vi "CatchSteer.vi"(6 "isOmni":bool, 8 "DefY":dbl, 9 "DefX":dbl, 10 "ReInit":bool) -> (0 "Translation X":dbl, 1 "Translation Y":dbl)   [LabVIEW 2013]
uses:
  Common Code/Change Detect Boolean.vi
  Robot Global Data.vi
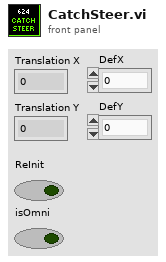
[diagram p1: front panel]
types:
  T1 = typedef "Vision Packet.ctl" = cluster{"Ball Found?":bool, "Ball X":dbl, "Ball Y":dbl, "Ball Diameter":dbl, "Gyro":dbl, "Vision Target":T2, "Timestamp":u32, "Camera":i16}
  T2 = typedef "Goal Info.ctl" = cluster{"Found?":bool, "Target Center":cluster{"X":dbl, "Y":dbl}, "Distance (ft)":dbl, "Hot?":bool, "Width":dbl, "Left?":bool}
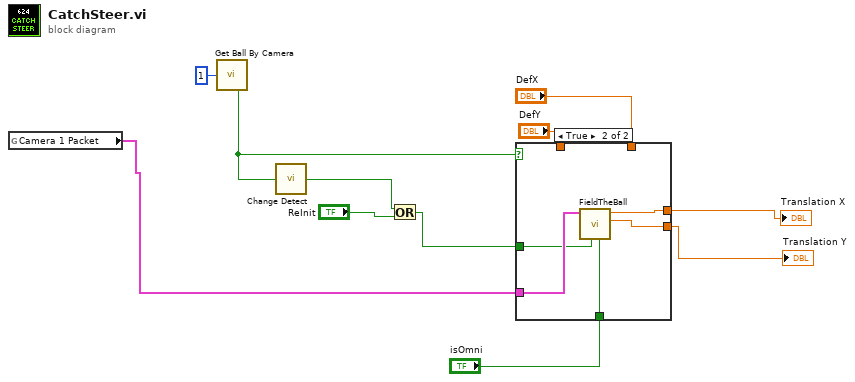
[diagram p0: block diagram]
diagram:
  n1 = global read "Robot Global Data.vi" "Camera 1 Packet"() -> (w3:T1)
  n2 = call "Get Ball By Camera.vi"("Camera"=i16 1) -> ("Ball Found?"=w2:bool)  [unwired: 9 in, 5 out]
  n3 = call-poly "Change Detect.vi"("In"=w2) -> ("Changed?"=w11:bool)
  n4 = Or(x=w11, y="ReInit") -> (x .or. y?=w9:bool)
  n5 = case shown="True" w2 {
    tunnel: w3 -> [_ w18]
    tunnel: [w13 w17] -> w4
    tunnel: w9 -> [_ w16]
    tunnel: "DefX" -> [w13 _]
    tunnel: [w12 w15] -> w5
    tunnel: "DefY" -> [w12 _]
    tunnel: "isOmni" -> [_ w14]
    frame False {
    }
    frame True {
      n6 = call "FieldTheBall.vi"("isOmni"=w14, "ReInit"=w16, "Original"=w18) -> ("Ty"=w15:dbl, "Tx"=w17:dbl)  [unwired: 7 in]
    }
  }
  "Translation X" <- w4
  "Translation Y" <- w5
